vi "Initialize.vi"(8 "error in (no error)":errorcluster, 11 "Sensor & Control in":refnum<class "Sensor & Control.lvclass">) -> (0 "error out":errorcluster, 3 "Sensor & Control out":refnum<class "Sensor & Control.lvclass">)   [LabVIEW 2013, in "Sensor & Control.lvib.lvlib" / "Sensor & Control.lvclass"]
uses:
  Sensor & Control.lvclass
  Sensor & Control.lvclass/Sensor & Control.ctl
  Read Setpoint.vi
  Read Value.vi
  Read Sampling Interval.vi
  Write VISA.vi
  <vilib>/Instr/_visa.llb/VISA Configure Serial Port (Instr).vi
  PluginInterface/PluginInterface.lvlibp/PluginInterfaceClass/Read Name.vi
  PluginInterface/PluginInterface.lvlibp/PluginInterfaceClass/Read TDMS File Path.vi
  PluginInterface/PluginInterface.lvlibp/PluginInterfaceClass/Read DVR.vi
  PluginInterface/PluginInterface.lvlibp/PluginInterfaceClass/Write TDMS.vi
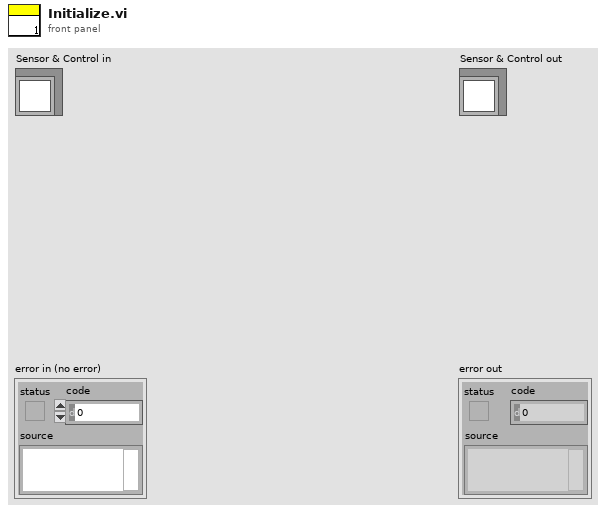
[diagram p1: front panel]
types:
  T1 = enum16{"open", "open or create", "create or replace", "create", "open (read-only)"}
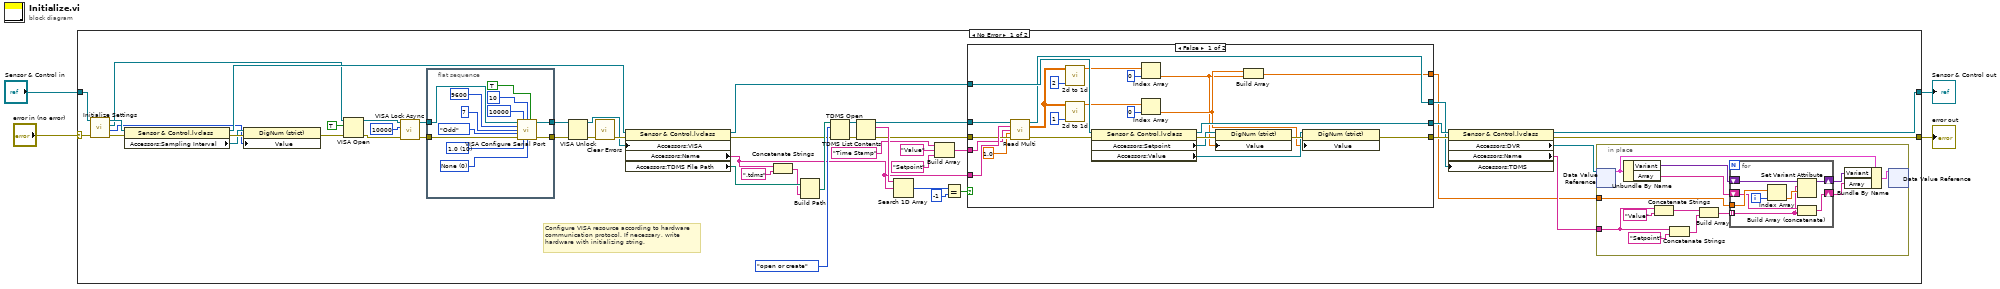
[diagram p0: block diagram]
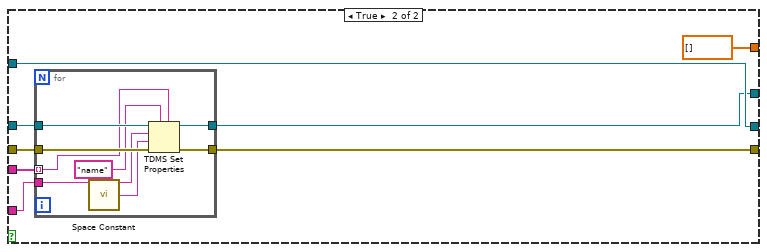
[diagram p2: hidden frame]
diagram:
  n1 = case shown="No Error" "error in (no error)" {
    selector: "error in (no error)" -> [w18 w128]
    tunnel: [w11 w128] -> w3
    tunnel: [w12 w127] -> w1
    tunnel: "Sensor & Control in" -> [w20 w127]
    frame No Error {
      # "Configure VISA resource according to hardware\ncommunication protocol. If necessary, write\nhardware with initializing string."
      n2 = call "Initialize Settings.vi"("error in (no error)"=w18, "Sensor & Control in"=w20) -> ("error out"=w13:errorcluster, "Sampling Interval 2"=w15:i32, "VISA out"=w17:refnum<visa-resource-name>, "Sensor & Control out"=w19:refnum<class "Sensor & Control.lvclass">)  [unwired: 6 in]
      n3 = property class="Sensor & Control.lvclass"(reference=w19, error in=w13) -> (reference out=w22:refnum<class "Sensor & Control.lvclass">, error out=w21:errorcluster, "Accessors:Sampling Interval"=w16:refnum<vi>)
      n4 = property class="DigNum (strict)"(reference=w16, error in=w21, "Value"=w15) -> (error out=w14:errorcluster)  [unwired: 1 out]
      n5 = VISA Open(duplicate session (F)=TRUE, error in (no error)=w14, VISA resource name=w17) -> (VISA resource name=w28:refnum<visa-resource-name>, error out=w31:errorcluster)  [unwired: 2 in]
      n6 = call <vilib>:"VISA Lock Async.vi"("error in (no error)"=w31, "timeout (0)"=u32 10000, "VISA resource name"=w28) -> ("error out"=w30:errorcluster, "VISA resource name out"=w29:refnum<visa-resource-name>)  [unwired: 6 in, 1 out]
      n7 = flat-sequence {
        tunnel: w29 -> [w81]
        tunnel: w30 -> [w80]
        tunnel: [w79] -> w26
        tunnel: [w78] -> w25
        frame #0 {
          w77 = u16 0 items=["None", "XON/XOFF", "RTS/CTS", "XON/XOFF & RTS/CTS", "DTR/DSR", "XON/XOFF & DTR/DSR"] ("flow control (0:none)")
          w83 = u16 10 items=["1.0"=10, "1.5"=15, "2.0"=20] ("stop bits (10: 1 bit)")
          n8 = call-poly "VISA Configure Serial Port"("VISA resource name"=w81, "timeout (10sec)"=u32 10000, "termination char\n(0xA = '\\n' = LF)"=u8 10 ("termination char\n(0xA = '\\n' = LF)"), "Enable Termination\nChar (T)"=TRUE ("Enable Termination\nChar (T)"), "baud rate (9600)"=u32 9600, "data bits (8)"=u16 7, "parity (0:none)"=enum16{"None", "Odd", "Even", "Mark", "Space"}."Odd", "error in (no error)"=w80, "stop bits (10: 1 bit)"=w83, "flow control (0:none)"=w77) -> ("VISA resource name out"=w78:refnum<visa-resource-name>, "error out"=w79:errorcluster)  [unwired: 4 out]
        }
      }
      n9 = VISA Unlock(8:w26, 11:w25) -> (0:w34:errorcluster, 3:w33:refnum<visa-resource-name>)
      n10 = call <vilib>:"Clear Errors.vi"("error in (no error)"=w34) -> ("error out"=w43:errorcluster)  [unwired: 6 in]
      n11 = property class="Sensor & Control.lvclass"(reference=w22, error in=w43, "Accessors:VISA"=w33) -> (reference out=w9:refnum<class "Sensor & Control.lvclass">, error out=w8:errorcluster, "Accessors:Name"=w10:string, "Accessors:TDMS File Path"=w39:path)
      n12 = Concatenate Strings(w10, ".tdms" ("name or relative path")) -> (w23:string)
      n13 = Build Path(base path=w39, name or relative path=w23) -> (appended path=w42:path)
      n14 = TDMS Open(8:w8, 10:T1."open or create" ("operation (0:open)"), 11:w42) -> (0:w41:errorcluster, 3:w38:refnum<k34>)  [unwired: 4 in]
      n15 = TDMS List Contents(4:w41, 7:w38) -> (0:w48:errorcluster, 2:w51:string[], 3:w49:refnum<k34>)  [unwired: 1 in, 1 out]
      n16 = Search 1D Array(1D array=w51, element=w10) -> (index of element=w52:i32)  [unwired: 1 in]
      n17 = Build Array("Time Stamp" ("Channel"), "Value" ("string"), "Setpoint" ("string")) -> (w47:string[])
      n18 = Equal?(x=w52, y=-1) -> (x = y?=w50:bool)
      n19 = case shown="False" w50 {
        tunnel: w49 -> [w103 w118]
        tunnel: [w93 w114] -> w37
        tunnel: w48 -> [w106 w116]
        tunnel: w10 -> [w107 w117]
        tunnel: w9 -> [w110 w113]
        tunnel: w47 -> [w91 w115]
        tunnel: [w102 w113] -> w36
        tunnel: [w90 w112] -> w32
        tunnel: [w87 dbl[] []] -> w6
        frame False {
          n20 = call "Read Multi.vi"("tdms file in"=w103, "group"=w107, "Channel"=w91, "Numeric"=1.0, "error in (no error)"=w106) -> ("tdms file out"=w90:refnum<k34>, "Array"=w100:dbl[][], "error out"=w105:errorcluster)  [unwired: 7 in, 1 out]
          n21 = call "2d to 1d.vi"("index"=2, "array"=w100) -> ("output array"=w108:dbl[])  [unwired: 9 in]
          n22 = call "2d to 1d.vi"("index"=1, "array"=w100) -> ("output array"=w99:dbl[])  [unwired: 9 in]
          n23 = property class="Sensor & Control.lvclass"(reference=w110, error in=w105) -> (reference out=w102:refnum<class "Sensor & Control.lvclass">, error out=w98:errorcluster, "Accessors:Setpoint"=w96:refnum<vi>, "Accessors:Value"=w92:refnum<vi>)
          n24 = Index Array(array=w108, index=0) -> (element=w88:dbl)
          n25 = Index Array(array=w99, index=0) -> (element=w89:dbl)
          n26 = property class="DigNum (strict)"(reference=w96, error in=w98, "Value"=w88) -> (error out=w97:errorcluster)  [unwired: 1 out]
          n27 = Build Array(w89, w88) -> (w87:dbl[])
          n28 = property class="DigNum (strict)"(reference=w92, error in=w97, "Value"=w89) -> (error out=w93:errorcluster)  [unwired: 1 out]
        }
        frame True {
          n29 = for {
            tunnel: w116 -> [w126]
            tunnel: [w125] -> w114
            tunnel: w118 -> [w124]
            tunnel: w117 -> [w123]
            tunnel: w115 -> [w122] mode=indexing
            tunnel: [w119] -> w112
            n30 = call <vilib>:"Space Constant.vi"() -> ("String"=w120:string)
            n31 = TDMS Set Properties(5:w122, 7:"name" ("property names"), 8:w126, 9:w120, 10:w123, 11:w124) -> (0:w125:errorcluster, 3:w119:refnum<k34>)  [unwired: 2 out]
          }
        }
      }
      n32 = property class="Sensor & Control.lvclass"(reference=w36, error in=w37, "Accessors:TDMS"=w32) -> (reference out=w12:refnum<class "Sensor & Control.lvclass">, error out=w11:errorcluster, "Accessors:DVR"=w5:refnum<data-value>, "Accessors:Name"=w7:string)
      n33 = in-place {
        in-place-border: w6 -> [w61]
        in-place-border: w7 -> [w58]
        n34 = in-place-dvr #1(w5) -> (w63:cluster{"Array":string[], "Variant":variant})  [unwired: 1 out]
        n35 = Unbundle By Name(w63) -> ("Variant"=w65:variant, "Array"=w55:string[])
        n36 = Concatenate Strings(w58, "Value" ("string")) -> (w57:string)
        n37 = Concatenate Strings(w58, "Setpoint" ("string")) -> (w56:string)
        n38 = Build Array(w57, w56) -> (w62:string[])
        n39 = for {
          tunnel: w62 -> [w68] mode=indexing
          tunnel: w61 -> [w71]
          shift-right: [w73] -> w64
          shift-left: w65 -> [w74]
          shift-right: [w67] -> w54
          shift-left: w55 -> [w69]
          i -> [w72]
          n40 = Index Array(array=w71, index=w72) -> (element=w70:dbl)
          n41 = Set Variant Attribute(Variant=w74, name=w68, value=w70) -> (Variant out=w73:variant)  [unwired: 1 in, 2 out]
          n42 = Build Array (concatenate)(w69, w68) -> (w67:string[])
        }
        n43 = Bundle By Name(cluster=w63, "Variant"=w64, "Array"=w54) -> (w66:cluster{"Array":string[], "Variant":variant})
        n44 = in-place-dvr #1(w66) -> ()  [unwired: 2 out]
      }
    }
    frame Error {
    }
  }
  "error out" <- w3
  "Sensor & Control out" <- w1
